vi "Process Output Queues.vi"(7 "tag bus queues":T19, 8 "error in":errorcluster, 10 "Outgoing Cyclic Cfg":T1 {"Outgoing Cyclic Frame"."Transmit Propreties"."Transmit Time" format="%#_p"}, 11 "J1939 internal data":T6={"J1939 XNET Settings"={"XNET Database"="", "XNET Cluster"="", "CAN port"="", "Baud rate [Bd]"=0, "J1939 Network Address"=0, "Name"=0, "Termination"=0}, "j1939 queues"={"Processed Outgoing"=refnum, "Process Outgoing"=refnum, "stop notifier"=refnum, "error queue"=refnum, "active dtc"=refnum, "processed inc"=refnum}, "fgv references"={"BAM Buffer"=refnum, "CM Buffer"=refnum, "CM Gen"=refnum, "BAM Gen"=refnum, "Address Claims"=refnum, "RQST"=refnum, "scaling lut"=refnum, "data lut"=refnum, "cyclic scheduler"=refnum}, "frame in"="", "frame out"="", "timing"={"tb to j1939 queue timeout"=100, "j1939 to tb queue timeout"=100, "dtc loop period (ms)"=100, "CAN in loop period (ms)"=100, "process incoming queue timeout (ms)"=100, "Outgoing Write Decimation"=0, "process outgoing loop rate (ms)"=0, "periodic outgoing queue timeout (ms)"=10, "CAN out queue timeout (ms)"=100}}) -> ()   [LabVIEW 2013, in "J1939.lvlib"]
uses:
  J1939.lvlib
  API Types/Tag Bus Queues.ctl
  <vilib>/NI/Tag Bus/table/data table.ctl
  API Types/Internal Data.ctl
  API Types/XNET Settings.ctl
  API Types/Setup Information Cluster.ctl
  API Types/CAN Outgoing Message Cluster.ctl
  API Types/Convert DTCs Cluster.ctl
  <vilib>/xnet/xnet.llb/XNET Frame CAN.ctl
  <vilib>/xnet/xnet.llb/XNET Frame Type CAN.ctl
  TP/TP List References.ctl
  BAM/BAM Buffer Connections List_Ref.ctl
  Connection Mode/Connection Mode Generation Connection Ref.ctl
  BAM/BAM Generation Connections List_Ref.ctl
  LUTs/J1939 Address Table Reference.ctl
  RQST/RQST Lookup Table Reference.ctl
  LUTs/J1939 Conversion Lookup Table Reference.ctl
  LUTs/J1939 Data Lookup Table Reference.ctl
  LUTs/Cyclic Frame Scheduler Lut Reference.ctl
  Configuration/TypeDefs/timing configuration.ctl
  CD/CD Outgoing Cyclic Configuration.ctl
  CD/CD Outgoing Cyclic Frame Pairs.ctl
  API Types/XNET Frame Event Properties.ctl
  module/configuration/Signal Mapping.ctl
  <vilib>/NI/Tag Bus/tag/Data Type.ctl
  <vilib>/NI/Tag Bus/table/data table.lvlib
  <vilib>/NI/Tag Bus/tag/tag descriptor.lvclass
  module/configuration/J1939 configuration.lvclass
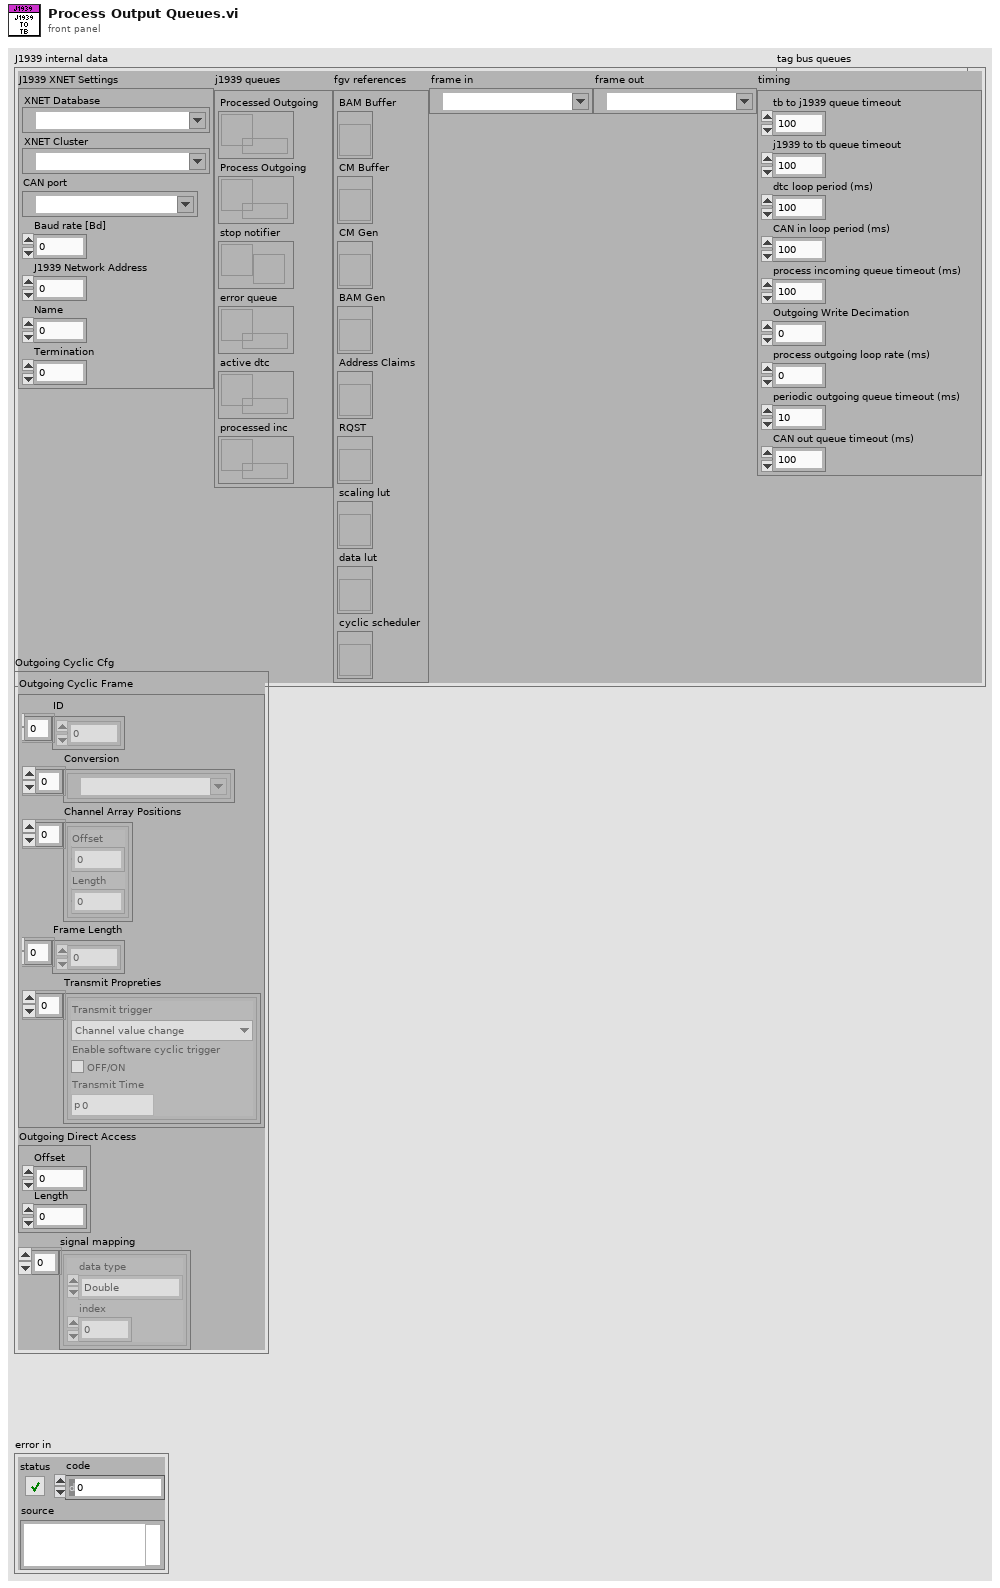
[diagram p1: front panel]
types:
  T1 = typedef "J1939.lvlib/CD Outgoing Cyclic Configuration.ctl" = cluster{"Outgoing Cyclic Frame":T2, "Outgoing Direct Access":cluster{"Offset":u32, "Length":u32}, "signal mapping":T4[]}
  T2 = typedef "J1939.lvlib/CD Outgoing Cyclic Frame Pairs.ctl" = cluster{"ID":u32[], "Conversion":refnum<k21>[], "Channel Array Positions":cluster{"Offset":u32, "Length":u32}[], "Frame Length":u32[], "Transmit Propreties":T3[]}
  T3 = typedef "J1939.lvlib/XNET Frame Event Properties.ctl" = cluster{"Transmit trigger":enum16{"Channel value change"}, "Enable software cyclic trigger":bool, "Transmit Time":dbl}
  T4 = typedef "J1939 configuration.lvclass/Signal Mapping.ctl" = cluster{"data type":T5, "index":i32}
  T5 = typedef "tag bus.lvlib/tag descriptor.lvclass/Data Type.ctl" = enum16{"Double", "Single", "I64", "I32", "I16", "I8", "U64", "U32", "U16", "U8", "Boolean", "String", "Array of Double", "Array of Single", "Array of I64", "Array of I32", "Array of I16", "Array of I8", "Array of U64", "Array of U32", "Array of U16", "Array of U8", "Array of Boolean", "Array of String"}
  T6 = typedef "J1939.lvlib/Internal Data.ctl" = cluster{"J1939 XNET Settings":T7, "j1939 queues":T8, "fgv references":T9, "frame in":refnum<k21>, "frame out":refnum<k21>, "timing":T18}
  T7 = typedef "J1939.lvlib/XNET settings.ctl" = cluster{"XNET Database":refnum<k21>, "XNET Cluster":refnum<k21>, "CAN port":refnum<k21>, "Baud rate [Bd]":u32, "J1939 Network Address":u8, "Name":u64, "Termination":u32}
  T8 = typedef "J1939.lvlib/Setup Information Cluster.ctl" = cluster{"Processed Outgoing":refnum<queue>, "Process Outgoing":refnum<queue>, "stop notifier":refnum<notifier>, "error queue":refnum<queue>, "active dtc":refnum<queue>, "processed inc":refnum<queue>}
  T9 = typedef "J1939.lvlib/TP List References.ctl" = cluster{"BAM Buffer":T10, "CM Buffer":T10, "CM Gen":T11, "BAM Gen":T12, "Address Claims":T13, "RQST":T14, "scaling lut":T15, "data lut":T16, "cyclic scheduler":T17}
  T10 = typedef "J1939.lvlib/BAM Buffer Connections List_Ref.ctl" = refnum<vi>
  T11 = typedef "J1939.lvlib/Connection Mode Generation Connection Ref.ctl" = refnum<vi>
  T12 = typedef "J1939.lvlib/BAM Generation Connections List_Ref.ctl" = refnum<vi>
  T13 = typedef "J1939.lvlib/J1939 Address Table Reference.ctl" = refnum<vi>
  T14 = typedef "J1939.lvlib/RQST Lookup Table Reference.ctl" = refnum<vi>
  T15 = typedef "J1939.lvlib/J1939 Conversion Lookup Table Reference.ctl" = refnum<vi>
  T16 = typedef "J1939.lvlib/J1939 Data Lookup Table Reference.ctl" = refnum<vi>
  T17 = typedef "J1939.lvlib/cyclic frame scheduler lut reference.ctl" = refnum<vi>
  T18 = typedef "J1939.lvlib/timing configuration.ctl" = cluster{"tb to j1939 queue timeout":i32, "j1939 to tb queue timeout":i32, "dtc loop period (ms)":i32, "CAN in loop period (ms)":i32, "process incoming queue timeout (ms)":i32, "Outgoing Write Decimation":u32, "process outgoing loop rate (ms)":i32, "periodic outgoing queue timeout (ms)":i32, "CAN out queue timeout (ms)":i32}
  T19 = typedef "J1939.lvlib/Tag Bus Queues.ctl" = cluster{"Input Queue (to background)":refnum<queue>, "Input Queue (from background)":refnum<queue>, "Output Queue (to background)":refnum<queue>, "Output Queue (from background)":refnum<queue>}
  T20 = typedef "tag bus.lvlib/data table.lvlib/data table.ctl" = cluster{"Double":dbl[], "Single":sgl[], "I64":i64[], "I32":i32[], "I16":i16[], "I8":i8[], "U64":u64[], "U32":u32[], "U16":u16[], "U8":u8[], "Boolean":bool[], "String":string[], "Array of Double":cluster{"DBL Array":dbl[]}[], "Array of Single":cluster{"SGL Array":sgl[]}[], "Array of I64":cluster{"I64 Array":i64[]}[], "Array of I32":cluster{"I32 Array":i32[]}[], "Array of I16":cluster{"I16 Array":i16[]}[], "Array of I8":cluster{"I8 Array":i8[]}[], "Array of U64":cluster{"U64 Array":u64[]}[], "Array of U32":cluster{"U32 Array":u32[]}[], "Array of U16":cluster{"U16 Array":u16[]}[], "Array of U8":cluster{"U8 Array":u8[]}[], "Array of Boolean":cluster{"Boolean Array":bool[]}[], "Array of String":cluster{"String Array":string[]}[]}
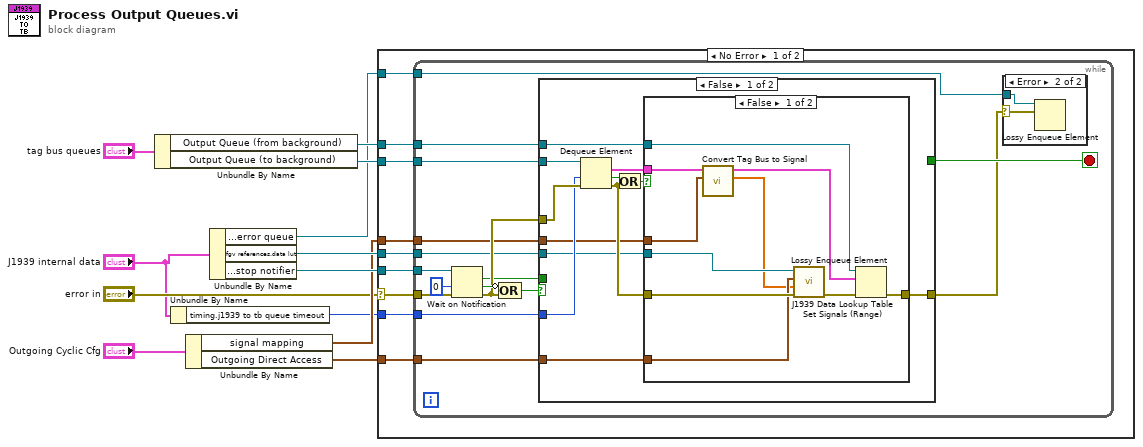
[diagram p0: block diagram]
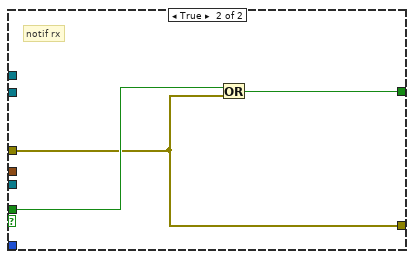
[diagram p4: hidden frame]
diagram:
  n1 = Unbundle By Name("tag bus queues") -> ("Output Queue (from background)"=w11:refnum<queue>, "Output Queue (to background)"=w12:refnum<queue>)
  n2 = Unbundle By Name("J1939 internal data") -> ("timing.j1939 to tb queue timeout"=w1:i32)
  n3 = Unbundle By Name("Outgoing Cyclic Cfg") -> ("signal mapping"=w8:T4[], "Outgoing Direct Access"=w5:cluster{"Offset":u32, "Length":u32})
  n4 = Unbundle By Name("J1939 internal data") -> ("j1939 queues.error queue"=w3:refnum<queue>, "fgv references.data lut"=w9:T16, "j1939 queues.stop notifier"=w10:refnum<notifier>)
  n5 = case shown="No Error" "error in" {
    selector: "error in" -> [w21 _]
    tunnel: w10 -> [w20 _]
    tunnel: w9 -> [w19 _]
    tunnel: w11 -> [w18 _]
    tunnel: w12 -> [w17 _]
    tunnel: w5 -> [w16 _]
    tunnel: w8 -> [w15 _]
    tunnel: w3 -> [w14 _]
    tunnel: w1 -> [w13 _]
    frame No Error {
      n6 = while {
        tunnel: w20 -> [w36]
        tunnel: w21 -> [w37]
        tunnel: w13 -> [w26]
        tunnel: w19 -> [w30]
        tunnel: w18 -> [w28]
        tunnel: w17 -> [w27]
        tunnel: w16 -> [w25]
        tunnel: w15 -> [w24]
        tunnel: w14 -> [w22]
        stop <- w31 stop-if-true
        n7 = Wait on Notification(notifier=w36, timeout in ms (-1)=0, error in (no error)=w37) -> (notification=w32:bool, timed out?=w35:bool, error out=w33:errorcluster)  [unwired: 1 in, 1 out]
        n8 = Compound Arithmetic op=OR(invert w35, w33) -> (w34:bool)
        n9 = case shown="False" w34 {
          tunnel: w33 -> [w51 w63]
          tunnel: w32 -> [_ w65]
          tunnel: [_ w64] -> w31
          tunnel: [w45 w63] -> w23
          tunnel: w30 -> [w42 _]
          tunnel: w28 -> [w43 _]
          tunnel: w27 -> [w50 _]
          tunnel: w26 -> [w49 _]
          tunnel: w25 -> [w41 _]
          tunnel: w24 -> [w40 _]
          frame False {
            n10 = Dequeue Element(queue=w50, timeout in ms (-1)=w49, error in (no error)=w51) -> (element=w46:T20, timed out?=w48:bool, error out=w44:errorcluster)  [unwired: 1 out]
            n11 = Or(x=w48, y=w44) -> (x .or. y?=w47:bool)
            n12 = case shown="False" w47 {
              tunnel: w46 -> [w53 _]
              tunnel: [w61 w62] -> w45
              tunnel: w44 -> [w58 w62]
              tunnel: w43 -> [w60 _]
              tunnel: w42 -> [w57 _]
              tunnel: w41 -> [w56 _]
              tunnel: w40 -> [w52 _]
              frame False {
                n13 = call "Convert Tag Bus to Signal.vi"("signal mapping"=w52, "data table in"=w53) -> ("Previous Chan Values out"=w55:dbl[], "data table out"=w54:T20)  [unwired: 8 in]
                n14 = call "J1939 Data Lookup Table Set Signals (Range).vi"("error in (no error)"=w58, "Signals"=w55, "Direct Access"=w56, "Ref in"=w57) -> ("error out"=w59:errorcluster)  [unwired: 6 in, 1 out]
                n15 = Lossy Enqueue Element(queue=w60, element=w54, error in (no error)=w59) -> (error out=w61:errorcluster)  [unwired: 3 out]
              }
              frame True {
              }
            }
          }
          frame True {
            # "notif rx"
            n16 = Or(x=w65, y=w63) -> (x .or. y?=w64:bool)
          }
        }
        n17 = case shown="Error" w23 {
          selector: w23 -> [_ w39]
          tunnel: w22 -> [_ w38]
          frame No Error {
          }
          frame Error {
            n18 = Lossy Enqueue Element(queue=w38, element=w39) -> ()  [unwired: 1 in, 4 out]
          }
        }
      }
    }
    frame Error {
    }
  }
